vi "Cohen_Kappa_Score.vi"(8 "error in (no error)":errorcluster caption="entrée d'erreur (pas d'erreur)", 9 "y2":string[][](array[string]), 10 "y1":string[][](array[string]), 11 "cohen_kappa_score":T1={"labels"=[], "weights"="None", "sample_weight"=[]}) -> (0 "error out":errorcluster caption="sortie d'erreur", 3 "Score":string)   [LabVIEW 2020]
doc: "Cohen’s kappa: a statistic that measures inter-annotator agreement.\n\nThis function computes Cohen’s kappa, a score that expresses the level of agreement between two annotators on a classification problem. It is defined as\n\nwhere is the empirical probability of agreement on the label assigned to any sample (the observed agreement ratio), and is the expected agreement when both annotators assign labels randomly. is estimated using a per-annotator empirical prior over the class labels.\n\n\n\nParameters : \n\n- y1 : array, shape = [n_samples]\nLabels assigned by the first annotator.\n\n- y2 : array, shape = [n_samples]\nLabels assigned by the second annotator. The kappa statistic is symmetric, so swapping y1 and y2 doesn’t change the value.\n\n- labels : array, shape = [n_classes], optional\nList of labels to index the matrix. This may be used to select a subset of labels. If None, all labels that appear at least once in y1 or y2 are used.\n\n- weights : str, optional\nWeighting type to calculate the score. None means no weighted; “linear” means linear weighted; “quadratic” means quadratic weighted.\n\n- sample_weight : array-like of shape (n_samples,), default=None\nSample weights.\n\nReturns : \n\n- kappa : float\nThe kappa statistic, which is a number between -1 and 1. The maximum value means complete agreement; zero or lower means chance agreement."
uses:
  Cohen_Kappa_Score.lvclass
panel:
  out "Cohen_Kappa_Score.lvclass":refnum<class "Cohen_Kappa_Score.lvclass">
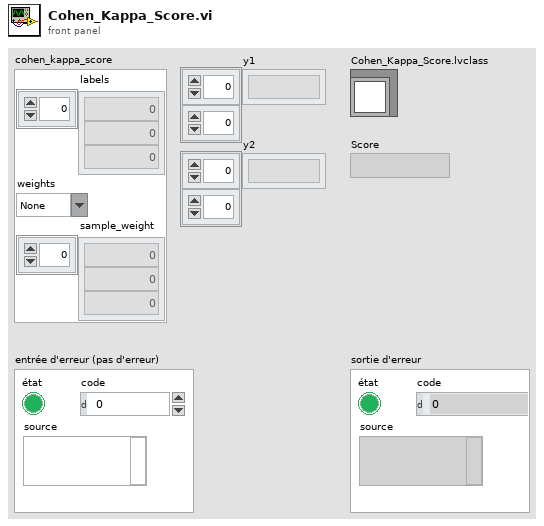
[diagram p1: front panel]
types:
  T1 = cluster{"labels":i32[], "weights":string, "sample_weight":dbl[]}
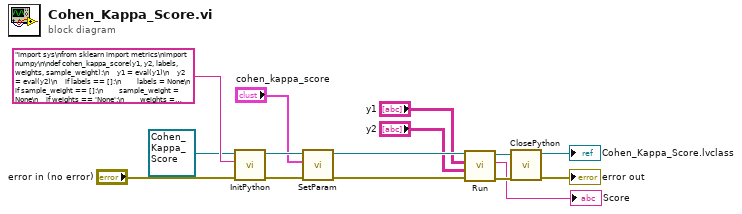
[diagram p0: block diagram]
diagram:
  n1 = call-dynamic "InitPython.vi"("error in (no error)"="error in (no error)", "Python Instruction"="import sys\nfrom sklearn import metrics\nimport numpy\n\ndef cohen_kappa_score(y1, y2, labels, weights, sample_weight):\n    y1 = eval(y1)\n    y2 = eval(y2)\n    if labels == []:\n        labels = None\n    if sample_weight == []:\n        sample_weight = None\n    if weights == 'None':\n        weights = None\n    try:\n        cohen_kappa_score = metrics.cohen_kappa_score(y1, y2, labels, weights, sample_weight)\n        cohen_kappa_score = cohen_kappa_score.tolist()\n        return str(cohen_kappa_score)\n    except:\n        erreur = sys.exc_info()\n        typerr = u\"%s\" % (erreur[0])\n        typerr = typerr[typerr.find(\"'\")+1:typerr.rfind(\"'\")]\n        msgerr = u\"%s\" % (erreur[1])\n        message = str('/!\\\\ {0} : {1}'. format(typerr,msgerr))\n        return message", "Scikit-learn en entrée"=refnum<class "Cohen_Kappa_Score.lvclass"> refnum ("Cohen_Kappa_Score.lvclass")) -> ("error out"=w10:errorcluster, "Scikit-learn en sortie"=w11:refnum<class "Cohen_Kappa_Score.lvclass">)  [unwired: 7 in]
  n2 = call-dynamic "SetParam.vi"("error in (no error)"=w10, "cohen_kappa_score"="cohen_kappa_score", "Cohen_Kappa_Score.lvclass"=w11) -> ("error out"=w7:errorcluster, "Cohen_Kappa_Score.lvclass"=w8:refnum<class "Cohen_Kappa_Score.lvclass">)  [unwired: 7 in]
  n3 = call-dynamic "Run.vi"("error in (no error)"=w7, "y2"="y2", "y1"="y1", "Cohen_Kappa_Score.lvclass"=w8) -> ("error out"=w5:errorcluster, "String Data"=→"Score":string, "Cohen_Kappa_Score.lvclass"=w6:refnum<class "Cohen_Kappa_Score.lvclass">)  [unwired: 5 in]
  n4 = call-dynamic "ClosePython.vi"("error in (no error)"=w5, "Scikit-learn en entrée"=w6) -> ("error out"=→"error out":errorcluster, "Scikit-learn en sortie"=→"Cohen_Kappa_Score.lvclass":refnum<class "Cohen_Kappa_Score.lvclass">)  [unwired: 8 in]
